vi "computeIncrementedString.vi"(10 "Input String":string, 11 "StringIncrement":refnum<class "StringIncrement.Alphabetical.lvclass">) -> (2 "Incremented String":string, 3 "StringIncrement out":refnum<class "StringIncrement.Alphabetical.lvclass">)   [LabVIEW 2013, in "UniqueName.lvlib" / "StringIncrement.Alphabetical.lvclass"]
uses:
  StringIncrement.Alphabetical.lvclass
  StringIncrement/StringIncrement.lvclass
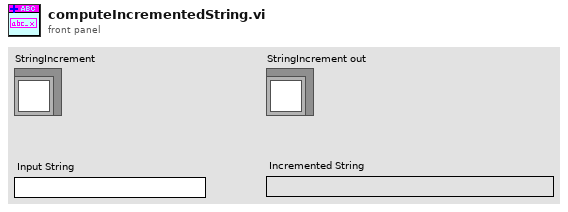
[diagram p1: front panel]
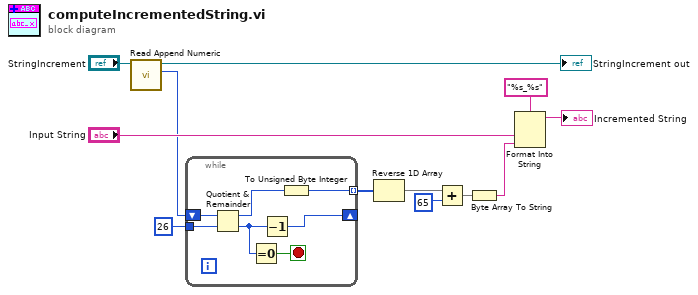
[diagram p0: block diagram]
diagram:
  n1 = call "Read Append Numeric.vi"("StringIncrement"="StringIncrement") -> ("Append Numeric"=w1:u32, "StringIncrement out"=→"StringIncrement out":refnum<class "StringIncrement.Alphabetical.lvclass">)  [unwired: 9 in]
  n2 = while {
    shift-right: [w14] -> _
    shift-left: w1 -> [w19]
    tunnel: [w13] -> w2 mode=indexing
    tunnel: u32 26 ("y") -> [w18]
    stop <- w17 stop-if-true
    n3 = Quotient & Remainder(x=w19, y=w18) -> (x-y*floor(x/y)=w16:u32, floor(x/y)=w15:u32)
    n4 = Equal To 0?(x=w15) -> (x = 0?=w17:bool)
    n5 = Decrement(x=w15) -> (x-1=w14:u32)
    n6 = To Unsigned Byte Integer(number=w16) -> (unsigned 8bit integer=w13:u8)
  }
  n7 = Reverse 1D Array(array=w2) -> (reversed array=w3:u8[])
  n8 = Add(x=w3, y=u8 65) -> (x+y=w5:u8[])
  n9 = Byte Array To String(unsigned byte array=w5) -> (string=w7:string)
  n10 = Format Into String(format string="%s_%s", "Input String", w7) -> (resulting string=→"Incremented String":string)  [unwired: 2 in, 1 out]
